vi "Send_UIWriteCtrlArray.vi"(7 "Value Signaling (F)":bool[](array[boolean]), 8 "error in":errorcluster, 9 "Control Data":variant[](array[variant]), 10 "Control Label":string[](array[string]), 11 "Queue in":refnum<queue>) -> (0 "error out":errorcluster)   [LabVIEW 2018, in "UI_Library.lvlib"]
uses:
  UI_Library.lvlib
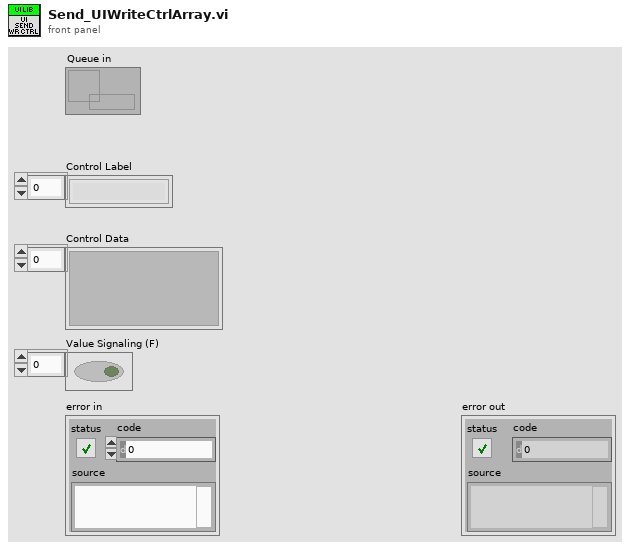
[diagram p1: front panel]
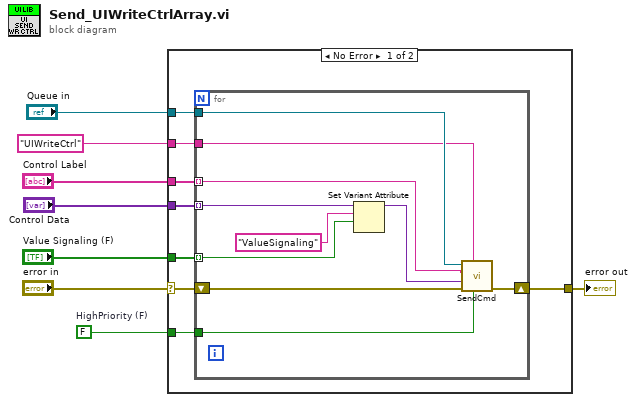
[diagram p0: block diagram]
diagram:
  w6 = FALSE  # HighPriority (F)
  n1 = case shown="No Error" "error in" {
    selector: "error in" -> [w15 w27]
    tunnel: "Queue in" -> [w16 _]
    tunnel: "Control Label" -> [w9 _]
    tunnel: "Control Data" -> [w11 _]
    tunnel: "UIWriteCtrl" ("UICmd") -> [w13 _]
    tunnel: w6 -> [w12 _]
    tunnel: [w14 w27] -> w8
    tunnel: "Value Signaling (F)" -> [w10 _]
    frame No Error {
      n2 = for {
        tunnel: w16 -> [w26]
        tunnel: w13 -> [w23]
        tunnel: w12 -> [w22]
        tunnel: w11 -> [w20] mode=indexing
        tunnel: w10 -> [w19] mode=indexing
        tunnel: w9 -> [w17] mode=indexing
        shift-right: [w24] -> w14
        shift-left: w15 -> [w25]
        n3 = Set Variant Attribute(Variant=w20, name="ValueSignaling", value=w19) -> (Variant out=w18:variant)  [unwired: 1 in, 2 out]
        n4 = call "SendCmd.vi"("HighPriority (F)"=w22, "UICmd"=w23, "error in"=w25, "Control Data"=w18, "Control Label"=w17, "Queue in"=w26) -> ("error out"=w24:errorcluster)  [unwired: 5 in]
      }
    }
    frame Error {
    }
  }
  "error out" <- w8
